vi "Write Numeric Range to Source (Base16 I16).vi"(4 "min":i16 format="%d bytes", 5 "<= max? (F)":bool, 6 "max":i16 format="%d bytes", 7 ">= min? (F)":bool, 8 "width (4)":i16=4, 9 "offset":i32, 10 "value":i16 format="%d bytes", 11 "error in":errorcluster) -> (1 "new offset":i32, 3 "error out":errorcluster)   [LabVIEW 2017, in "Static Errors.lvlib"]
doc: "Writes a string in the form of <b>min</b> <=/< <b>value</b> <=/< <b>max</b> to the source string of the provided <b>error cluster</b> at the specified <b>offset</b>."
uses:
  Static Errors.lvlib
  Write Numeric Scalar to Source (Base16 I16).vi
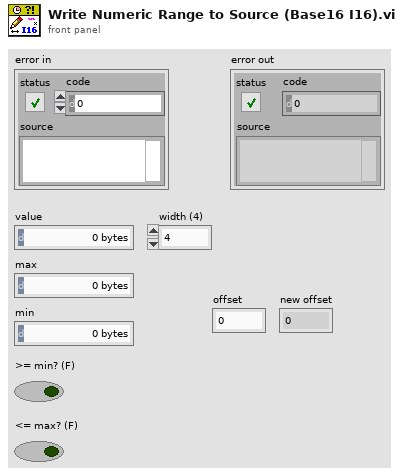
[diagram p1: front panel]
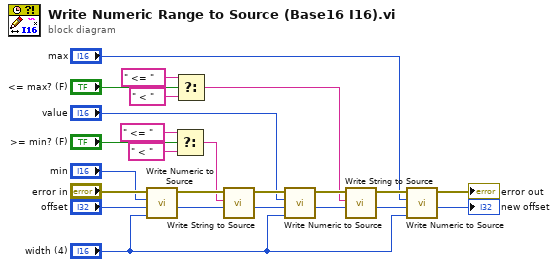
[diagram p0: block diagram]
diagram:
  n1 = call-poly "Write Numeric to Source.vi"("width (4)"="width (4)", "offset"="offset", "value"="min", "error in"="error in") -> ("new offset"=w23:i32, "error out"=w24:errorcluster)  [unwired: 6 in]
  n2 = Select(t=" <= ", s=">= min? (F)", f=" < ") -> (s? t:f=w8:string)
  n3 = Select(t=" <= ", s="<= max? (F)", f=" < ") -> (s? t:f=w2:string)
  n4 = call "Write String to Source.vi"("offset"=w23, "string"=w8, "error in"=w24) -> ("new offset"=w21:i32, "error out"=w22:errorcluster)  [unwired: 7 in]
  n5 = call-poly "Write Numeric to Source.vi"("width (4)"="width (4)", "offset"=w21, "value"="value", "error in"=w22) -> ("new offset"=w19:i32, "error out"=w20:errorcluster)  [unwired: 6 in]
  n6 = call "Write String to Source.vi"("offset"=w19, "string"=w2, "error in"=w20) -> ("new offset"=w17:i32, "error out"=w18:errorcluster)  [unwired: 7 in]
  n7 = call-poly "Write Numeric to Source.vi"("width (4)"="width (4)", "offset"=w17, "value"="max", "error in"=w18) -> ("new offset"=→"new offset":i32, "error out"=→"error out":errorcluster)  [unwired: 6 in]
